vi "寻最大值位置.vi"(8 "步进":dbl, 9 "起点":dbl, 11 "数据":dbl[](array[numeric]) caption="X") -> (1 "Amplitudes":dbl caption="振幅", 3 "position":dbl)   [LabVIEW 2016]
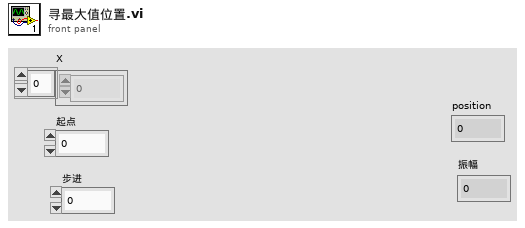
[diagram p1: front panel]
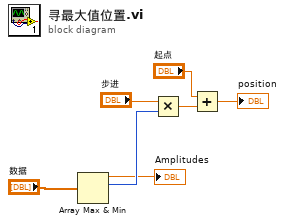
[diagram p0: block diagram]
diagram:
  n1 = Array Max & Min(array="数据") -> (max value=→"Amplitudes":dbl, max index (indices)=w3:i32)  [unwired: 2 out]
  n2 = Multiply(x="步进", y=w3) -> (x*y=w6:dbl)
  n3 = Add(x="起点", y=w6) -> (x+y=→"position":dbl)
